vi "CleanUp.vi"(8 "error in (no error)":errorcluster, 11 "Object in":refnum<class "SoldOutState.lvclass">) -> (0 "error out":errorcluster, 3 "object out":refnum<class "SoldOutState.lvclass">)   [LabVIEW 2020, in "SoldOutState.lvclass"]
uses:
  SoldOutState.lvclass
  State_class/State.lvclass
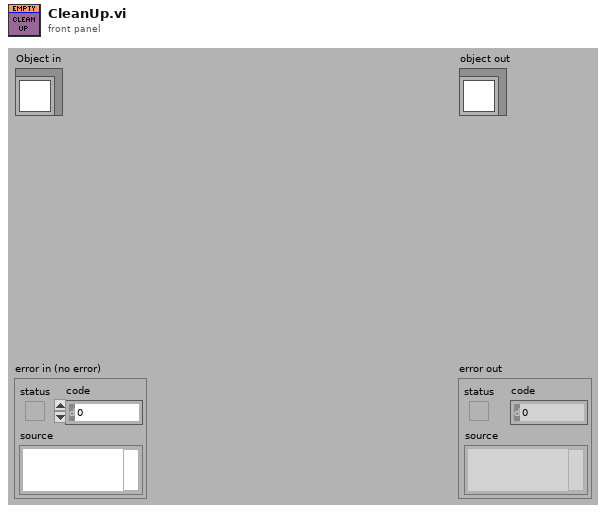
[diagram p1: front panel]
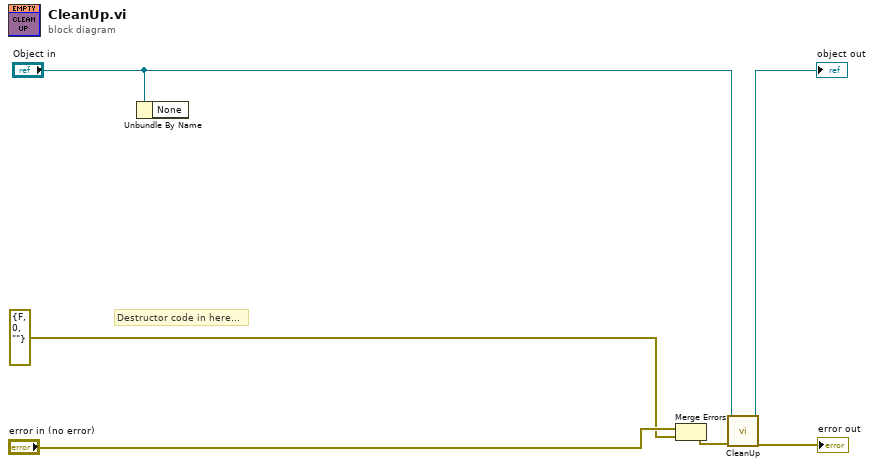
[diagram p0: block diagram]
diagram:
  # "Destructor code in here..."
  n1 = Unbundle By Name("Object in") -> ()  [unwired: 1 out]
  n2 = Merge Errors("error in (no error)", errorcluster {"status"=FALSE, "code"=0, "source"=""} ("error in (no error)")) -> (w2:errorcluster)
  n3 = call-parent "CleanUp.vi"("error in (no error)"=w2, "object in"="Object in") -> ("error out"=→"error out":errorcluster, "object out"=→"object out":refnum<class "SoldOutState.lvclass">)  [unwired: 8 in]
